vi "Initialize Switch.vi"(8 "Location":T1, 11 "Switch Unit In":T2=enum."Pickering") -> (0 "Initialization Failed!!":bool, 3 "Switch Unit":T2=enum."Pickering")   [LabVIEW 2022 SP3]
uses:
  SwitchOption.ctl
  -ScanSystem/Controls/location.ctl
  SwitchGlobals.vi
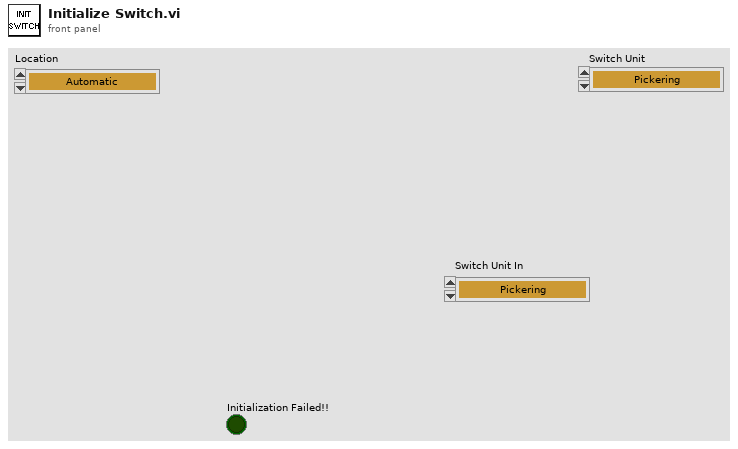
[diagram p1: front panel]
types:
  T1 = typedef "location.ctl" = enum16{"Automatic", "WCM Main", "Hawaii", "Columbia MM3000", "Columbia  NI System", "NYU", "RRI 2", "UHI Allen", "CUMC RT", "Chiba", "Stony Brook", "WCM Microscopy", "WCM Aeoretch", "WCM Optics Lab", "WCM Main 2Axis", "WCM Rotation", "WCM SAM SMAC", "SERI GP"}
  T2 = typedef "SwitchOption.ctl" = enum16{"Cytex", "Pickering", "NI Switch", "No Switch", "Riverside USB"}
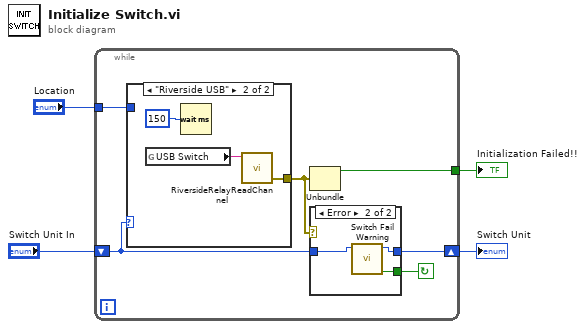
[diagram p0: block diagram]
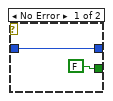
[diagram p2: hidden frame]
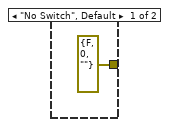
[diagram p3: hidden frame]
diagram:
  n1 = while {
    shift-right: [w8] -> w3
    shift-left: "Switch Unit In" -> [w9]
    tunnel: [w6] -> w2
    tunnel: "Location" -> [w5]
    stop <- w10 continue-if-true
    n2 = case shown="\"Riverside USB\"" w9 {
      tunnel: [errorcluster {"status"=FALSE, "code"=0, "source"=""} ("error out") w19] -> w7
      tunnel: w5 -> [_ _]
      frame "No Switch", Default {
      }
      frame "Riverside USB" {
        n3 = global read "SwitchGlobals.vi" "USB Switch"() -> (w17:string)
        n4 = Wait (ms)(milliseconds to wait=u32 150) -> ()  [unwired: 1 out]
        n5 = call "RiversideRelayReadChannel.vi"("serial_number"=w17) -> ("error out"=w19:errorcluster)  [unwired: 5 in, 1 out]
      }
    }
    n6 = Unbundle(w7) -> ("status"=w6:bool)  [unwired: 2 out]
    n7 = case shown="Error" w7 {
      tunnel: w9 -> [w12 w15]
      tunnel: [w12 w14] -> w8
      tunnel: [FALSE ("Retry") w13] -> w10
      frame No Error {
      }
      frame Error {
        n8 = call "Switch Fail Warning.vi"("Switch Unit"=w15) -> ("Retry"=w13:bool, "Switch Unit"=w14:T2)  [unwired: 9 in]
      }
    }
  }
  "Switch Unit" <- w3
  "Initialization Failed!!" <- w2
